vi "Get Lowest Target.vi"(11 "Target Info":T1(array[cluster])) -> (3 "Cluster":T2)   [LabVIEW 2011]
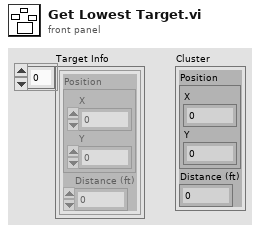
[diagram p1: front panel]
types:
  T1 = cluster{"Position":cluster{"X":dbl, "Y":dbl}, "Distance (ft)":dbl}[]
  T2 = cluster{"Position":cluster{"X":dbl, "Y":dbl}, "Distance (ft)":dbl}
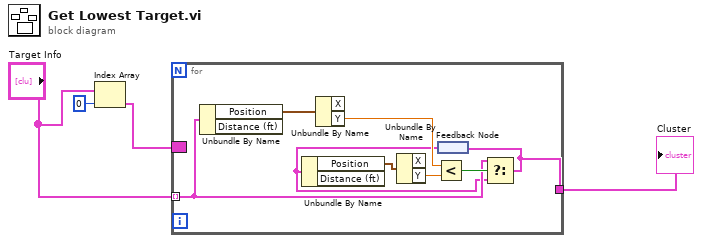
[diagram p0: block diagram]
diagram:
  n1 = Index Array(array="Target Info", index=0) -> (element=w3:T2)
  n2 = for {
    tunnel: "Target Info" -> [w7] mode=indexing
    border: w3 -> [_]
    tunnel: [w5] -> w4
    n3 = Unbundle By Name(w7) -> ("Position"=w12:cluster{"X":dbl, "Y":dbl})  [unwired: 1 out]
    n4 = Unbundle By Name(w12) -> ("Y"=w9:dbl)  [unwired: 1 out]
    n5 = feedback #1() -> (w6:T2)
    n6 = Unbundle By Name(w6) -> ("Position"=w11:cluster{"X":dbl, "Y":dbl})  [unwired: 1 out]
    n7 = Unbundle By Name(w11) -> ("Y"=w8:dbl)  [unwired: 1 out]
    n8 = Less?(x=w9, y=w8) -> (x < y?=w10:bool)
    n9 = Select(t=w7, s=w10, f=w6) -> (s? t:f=w5:T2)
    n10 = feedback-in #1(w5) -> ()
  }
  "Cluster" <- w4
